vi "Write Channel Names.vi"(8 "error in (no error)":errorcluster, 10 "Channel Names":string[](array[string])=["Telescope RA", "Telescope DEC", "Telescope Moving?", "Telescope Status"], 11 "Telescope in":refnum<class "Telescope.lvclass">) -> (0 "error out":errorcluster, 3 "Telescope out":refnum<class "Telescope.lvclass">)   [LabVIEW 2022 SP3, in "Telescope.lvclass"]
uses:
  Telescope.lvclass
  Telescope.lvclass/Telescope.ctl
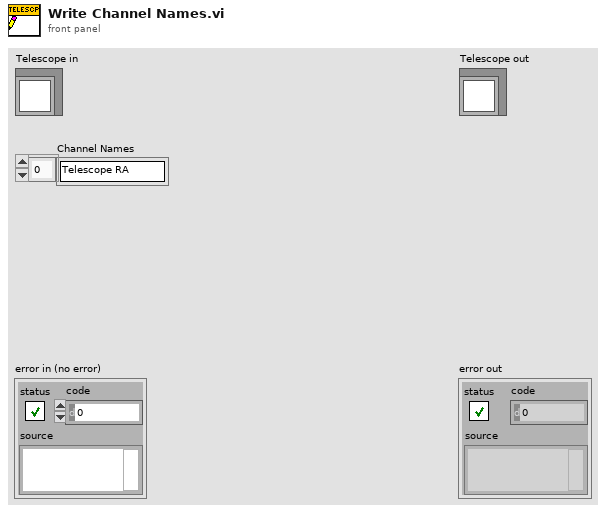
[diagram p1: front panel]
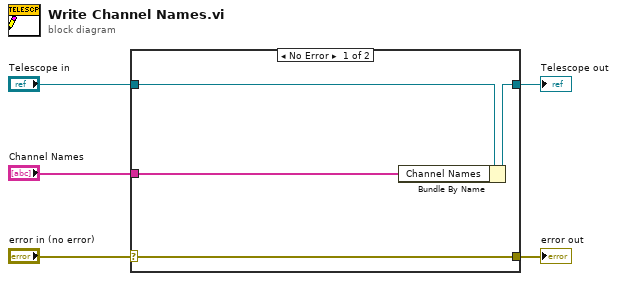
[diagram p0: block diagram]
diagram:
  n1 = case shown="No Error" "error in (no error)" {
    selector: "error in (no error)" -> [w9 w10]
    tunnel: [w9 w10] -> w4
    tunnel: [w7 w11] -> w2
    tunnel: "Telescope in" -> [w8 w11]
    tunnel: "Channel Names" -> [w6 _]
    frame No Error {
      n2 = Bundle By Name(cluster=w8, "Channel Names"=w6) -> (w7:refnum<class "Telescope.lvclass">)
    }
    frame Error {
    }
  }
  "error out" <- w4
  "Telescope out" <- w2
